vi "G#Object_EnableDebug.vi"(0 "set (F)":bool, 2 "debug enable (F)":bool, 5 "error in (no error)":errorcluster) -> (14 "already enabled":bool, 16 "enabled":bool, 19 "error out":errorcluster)   [LabVIEW 2017, in "G#Object.lvclass"]
doc: "Sets if debug is enabled. This means that methods could be executed as top level VIs and will create an object if needed. This is very useful when developing methods and testing them isolated."
uses:
  G#Object.lvclass
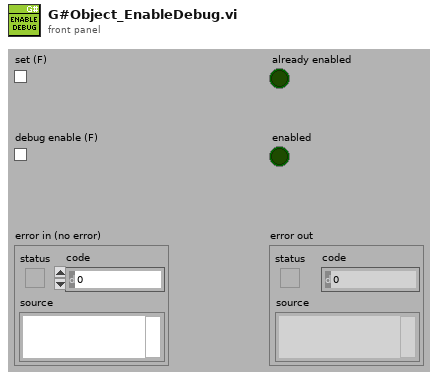
[diagram p1: front panel]
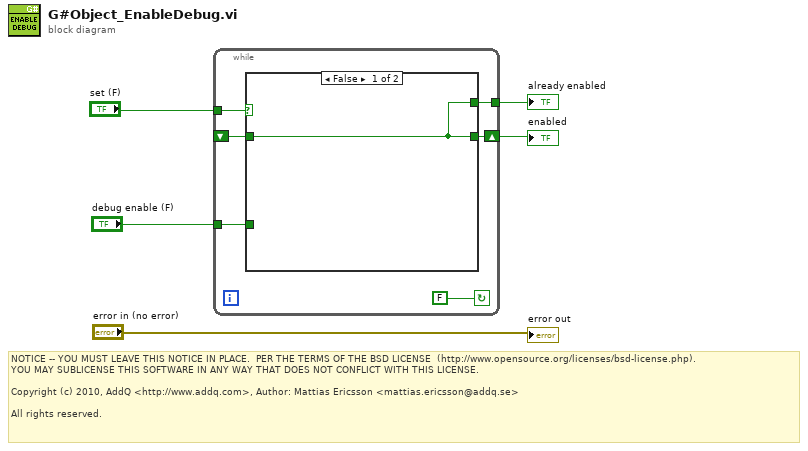
[diagram p0: block diagram]
diagram:
  # "NOTICE -- YOU MUST LEAVE THIS NOTICE IN PLACE.  PER THE TERMS OF THE BSD LICENSE  (http://www.opensource.org/licenses/bsd-license.php).\nYOU MAY SUBLICENSE THIS SOFTWARE IN ANY WAY THAT DOES NOT CONFLICT WITH THIS LICENSE.\n\nCopyright (c) 2010, AddQ <http://www.addq.com>, Author: Mattias Ericsson <mattias.ericsson@addq.se>\n\nAll rights reserved."
  n1 = while {
    shift-right: [w10] -> w5
    shift-left: _ -> [w8]
    tunnel: "set (F)" -> [w11]
    tunnel: "debug enable (F)" -> [w9]
    tunnel: [w6] -> w4
    stop <- FALSE continue-if-true
    n2 = case shown="False" w11 {
      tunnel: [w12 w14] -> w10
      tunnel: w9 -> [_ w14]
      tunnel: w8 -> [w12 w13]
      tunnel: [w12 w13] -> w6
      frame False {
      }
      frame True {
      }
    }
  }
  "enabled" <- w5
  "already enabled" <- w4
  "error out" <- "error in (no error)"
